vi "Init_Stage.vi"(7 "Settings":T1, 8 "error in (no error)":errorcluster, 9 "Long Travel Stage":refnum<k24>, 10 "Tools.wpf":refnum<k24>, 11 "ThorlabsLTS in":refnum<class "ThorlabsLTS.lvclass">) -> (0 "error out":errorcluster, 2 "Serial Number":string="83841487", 3 "ThorlabsLTS out":refnum<class "ThorlabsLTS.lvclass">)   [LabVIEW 2020, in "ThorlabsLTS.lvclass"]
uses:
  ThorlabsLTS.lvclass
  C:/GEECS/Developers Version/builds/Device builds/ThorLabsLTS/Thorlabs.MotionControl.Tools.WPF.UI.dll
  Thorlabs.MotionControl.Tools.WPF.UI.dll
  C:/GEECS/Developers Version/builds/Device builds/ThorLabsLTS/Thorlabs.MotionControl.Controls.dll
  Thorlabs.MotionControl.Controls.dll
  settingsThorlabsLTS_TypDef.ctl
  source/Device Drivers/shared/numericVariable_TypeDef.ctl
  C:/GEECS/Developers Version/builds/Device builds/ThorLabsLTS/Thorlabs.MotionControl.IntegratedStepperMotorsCLI.dll
  Thorlabs.MotionControl.IntegratedStepperMotorsCLI.dll
  ThorlabsLTS.lvclass/ThorlabsLTS.ctl
  source/Device Drivers/BaseDriver/BaseDriver.lvclass
panel:
  out "CreateDevice":bool
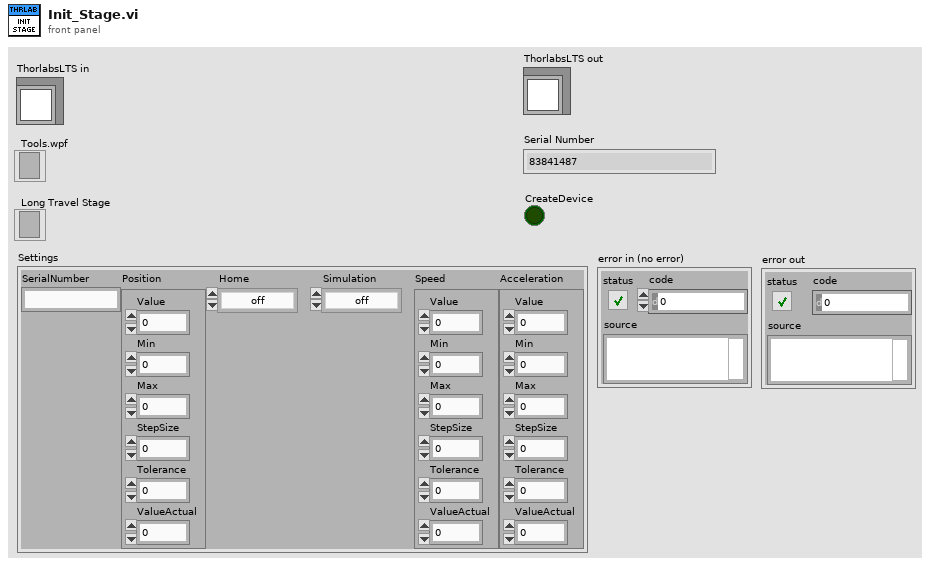
[diagram p1: front panel]
types:
  T1 = typedef "ThorlabsLTS.lvclass/settingsThorlabsLTS_TypDef.ctl" = cluster{"SerialNumber":string, "Position":T2, "Home":enum16{"off", "on"}, "Simulation":enum16{"off", "on"}, "Speed":T2, "Acceleration":T2}
  T2 = typedef "BaseDriver.lvclass/numericVariable_TypeDef.ctl" = cluster{"Value":dbl, "Min":dbl, "Max":dbl, "StepSize":dbl, "Tolerance":dbl, "ValueActual":dbl}
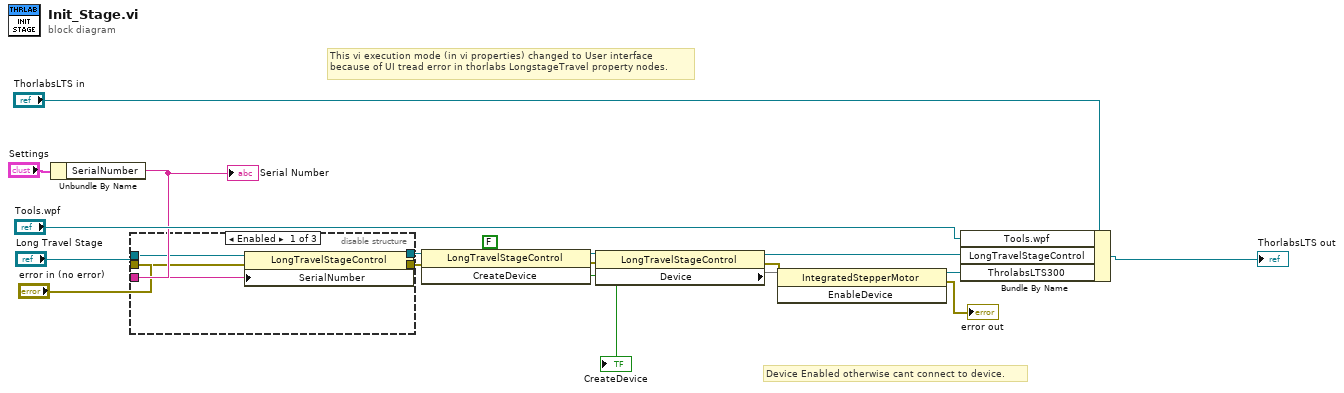
[diagram p0: block diagram]
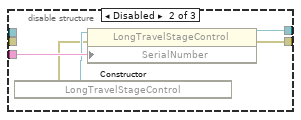
[diagram p2: hidden frame]
diagram:
  (unwired) FALSE ("CreateDevice")
  # "Device Enabled otherwise cant connect to device."
  # "This vi execution mode (in vi properties) changed to User interface\nbecause of UI tread error in thorlabs LongstageTravel property nodes."
  n1 = Unbundle By Name("Settings") -> ("SerialNumber"=w8:string)
  "Serial Number" <- w8
  n2 = disable-structure shown="Enabled" {
    disable-tunnel: "Long Travel Stage" -> [w22 _ _]
    disable-tunnel: [w21 w27 _] -> w15
    disable-tunnel: w8 -> [w20 w26 _]
    disable-tunnel: [w19 w25 _] -> w7
    disable-tunnel: "error in (no error)" -> [w18 _ _]
    frame Enabled {
      n3 = property class="LongTravelStageControl"(reference=w22, error in=w18, "SerialNumber"=w20) -> (reference out=w21:refnum<k24>, error out=w19:errorcluster)
    }
    frame Disabled {
      n4 = constructor class="Thorlabs.MotionControl.Controls"() -> (reference out=w24:refnum<k24>, error out=w23:errorcluster)  [unwired: 3 in, 1 out]
      n5 = property class="LongTravelStageControl"(reference=w24, error in=w23, "SerialNumber"=w26) -> (reference out=w27:refnum<k24>, error out=w25:errorcluster)
    }
    frame Disabled {
    }
  }
  n6 = invoke class="LongTravelStageControl" method="CreateDevice"(reference=w15, error in=w7) -> (reference out=w5:refnum<k24>, error out=w6:errorcluster, "CreateDevice"=→"CreateDevice":bool)  [unwired: 1 in]
  n7 = property class="LongTravelStageControl"(reference=w5, error in=w6) -> (reference out=w13:refnum<k24>, error out=w11:errorcluster, "Device"=w10)
  n8 = invoke class="IntegratedStepperMotor" method="EnableDevice"(reference=w10, error in=w11) -> (reference out=w14:refnum<k24>, error out=→"error out":errorcluster)  [unwired: 1 in, 1 out]
  n9 = Bundle By Name(cluster="ThorlabsLTS in", "Tools.wpf"="Tools.wpf", "LongTravelStageControl"=w13, "ThrolabsLTS300"=w14) -> (→"ThorlabsLTS out":refnum<class "ThorlabsLTS.lvclass">)
